vi "#2_MAV_MSG_SYS_TIME.vi"(11 "mavlink_payload":u8[](array[numeric])) -> (3 "SYSTEM_TIME":T1)   [LabVIEW 2023]
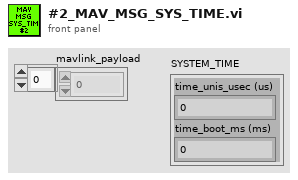
[diagram p1: front panel]
types:
  T1 = cluster{"time_unis_usec (us)":u64, "time_boot_ms (ms)":u32}
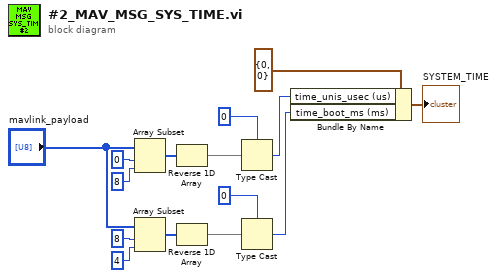
[diagram p0: block diagram]
diagram:
  n1 = Array Subset(array="mavlink_payload", index=0, length=8) -> (w14:u8[])
  n2 = Array Subset(array="mavlink_payload", index=8 ("length"), length=4) -> (w13:u8[])
  n3 = Reverse 1D Array(array=w14) -> (reversed array=w15:u8[])
  n4 = Reverse 1D Array(array=w13) -> (reversed array=w7:u8[])
  n5 = Type Cast(type=u64 0 ("index"), x=w15) -> (*(type *) &x=w4:u64)
  n6 = Type Cast(type=u32 0 ("index"), x=w7) -> (*(type *) &x=w3:u32)
  n7 = Bundle By Name(cluster=T1 {"time_unis_usec (us)"=0, "time_boot_ms (ms)"=0} ("System Time"), "time_unis_usec (us)"=w4, "time_boot_ms (ms)"=w3) -> (→"SYSTEM_TIME":T1)
